vi "ex6-10.vi"   [LabVIEW 2013]
uses:
  <vilib>/NXT/Block Support/NXT_InputPort.ctl
  <vilib>/NXT/Subs/MotorOutput.ctl
  <vilib>/NXT/Dual Mode Library/Logging/LogRedData_light.vi
  <vilib>/NXT/Dual Mode Library/Motors/MotorBrake.vi
  <vilib>/NXT/Dual Mode Library/Waits/Wait_Num.vi
  <vilib>/NXT/Dual Mode Library/Motors/MotorOn.vi
types:
  T1 = typedef "MotorOutput.ctl" = u8
  T2 = typedef "NXT_InputPort.ctl" = u32
  T3 = cluster{"Sample Time (0.5 sec)":sgl, "Time (10 sec)":sgl}
  T4 = typedef "LVHSConnector.ctl" = refnum<class "BrickReference.lvclass">
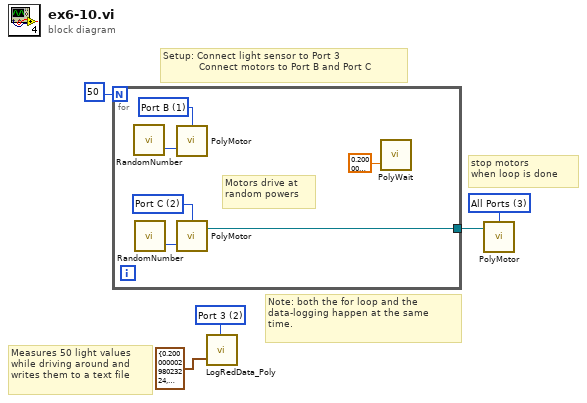
[diagram p0: block diagram]
diagram:
  w5 = T1 3 items=["Port A"=0, "Port B"=1, "Port C"=2, "Ports A & B"=4, "Ports A & C"=5, "Ports B & C"=6, "All Ports"=3] ("Port (All Ports)")
  w2 = T2 2 items=["Port 1", "Port 2", "Port 3", "Port 4"] ("Port (Port 3)")
  # "stop motors\nwhen loop is done"
  # "Note: both the for loop and the\ndata-logging happen at the same\ntime."
  # "Measures 50 light values\nwhile driving around and\nwrites them to a text file"
  # "Setup: Connect light sensor to Port 3\n            Connect motors to Port B and Port C"
  n1 = for {
    N: i16 50 ("Time (10 sec)") -> [_]
    tunnel: [w8] -> w4
    w6 = T1 2 items=["Port A"=0, "Port B"=1, "Port C"=2, "Ports A & B"=4, "Ports A & C"=5, "Ports B & C"=6, "All Ports"=3] ("Output Port (All Ports)")
    w7 = T1 1 items=["Port A"=0, "Port B"=1, "Port C"=2, "Ports A & B"=4, "Ports A & C"=5, "Ports B & C"=6, "All Ports"=3] ("Output Port (All Ports)")
    # "Motors drive at\nrandom powers"
    n2 = call <vilib>:"RandomNumber.vi"() -> ("Random Number"=w10:u16)  [unwired: 3 in, 1 out]
    n3 = call <vilib>:"RandomNumber.vi"() -> ("Random Number"=w9:u16)  [unwired: 3 in, 1 out]
    n4 = call-poly <vilib>:"PolyMotor.vi"("Power (75)"=w10, "Output Port (All Ports)"=w7) -> ()  [unwired: 1 in, 2 out]
    n5 = call-poly <vilib>:"PolyMotor.vi"("Power (75)"=w9, "Output Port (All Ports)"=w6) -> ("NXT/EV3"=w8:T4)  [unwired: 1 in, 1 out]
    n6 = call-poly <vilib>:"PolyWait.vi"("Time (1 sec)"=sgl 0.2 ("Time (sec)")) -> ()  [unwired: 1 in, 3 out]
  }
  n7 = call-poly <vilib>:"LogRedData_Poly.vi"("Parameters"=T3 {"Sample Time (0.5 sec)"=0.2, "Time (10 sec)"=10.0}, "Port (Port 3)"=w2) -> ()  [unwired: 1 in, 2 out]
  n8 = call-poly <vilib>:"PolyMotor.vi"("NXT/EV3"=w4, "Port (All Ports)"=w5) -> ()  [unwired: 3 out]
